vi "限幅滤波.vi"() -> ()   [LabVIEW 2015]
panel:
  out "x/y":dbl
  in  "幅值":i32
  in  "实时采样值":i32
  in  "stop":bool
  in  "采样数":i32
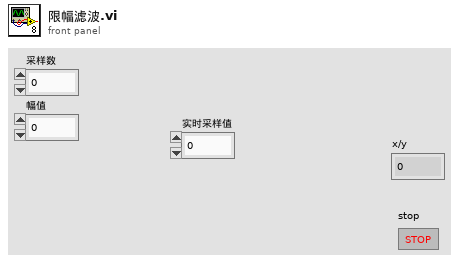
[diagram p1: front panel]
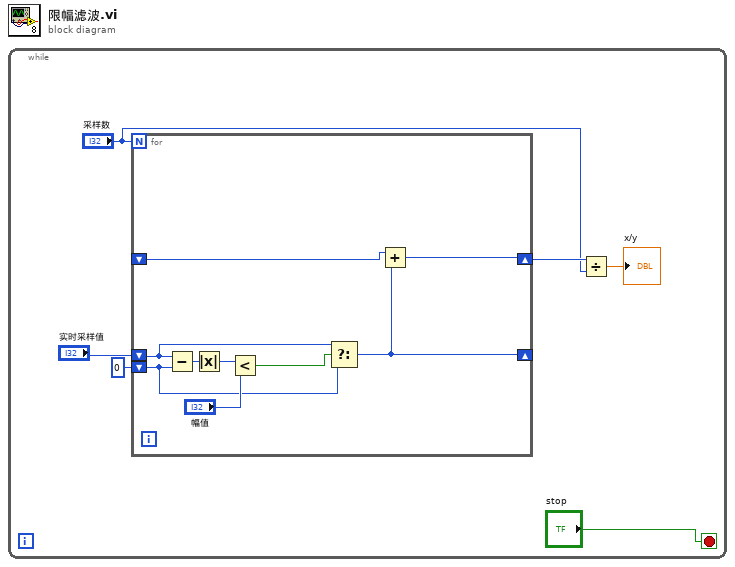
[diagram p0: block diagram]
diagram:
  n1 = while {
    stop <- "stop" stop-if-true
    n2 = for {
      N: "采样数" -> [_]
      shift-right: [w8] -> w4
      shift-left: _ -> [w9]
      shift-right: [w10] -> _
      shift-left: "实时采样值" -> [w12]
      shift-left: 0 ("实时采样值") -> [w11]
      n3 = Subtract(x=w12, y=w11) -> (x-y=w15:i32)
      n4 = Absolute Value(x=w15) -> (abs(x)=w7:i32)
      n5 = Less?(x=w7, y="幅值") -> (x < y?=w13:bool)
      n6 = Select(t=w12, s=w13, f=w11) -> (s? t:f=w10:i32)
      n7 = Add(x=w9, y=w10) -> (x+y=w8:i32)
    }
    n8 = Divide(x=w4, y="采样数") -> (x/y=→"x/y":dbl)
  }
